vi "ParamClusterControlCore.vi"(7 "timeout in ms (100ms)":i32=100, 8 "IO queue":refnum<queue>, 9 "SetGetCommands":string[][](array[string]), 10 "Command queue":refnum<queue>, 11 "Cluster ref":refnum<vi>) -> ()   [LabVIEW 2021]
uses:
  <vilib>/Utility/Data Type/NI_Data Type.lvlib
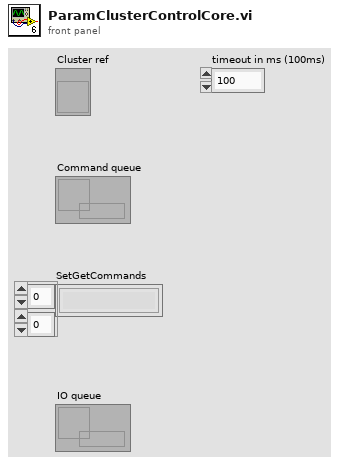
[diagram p1: front panel]
types:
  T1 = cluster{"Operation":enum16{"read", "write"}, "Data":string, "Queue":refnum<queue>}
  T2 = typedef "NI_Data Type.lvlib/Data Type.ctl" = enum8{"Invalid Type", "Void", "I8", "I16", "I32", "I64", "U8", "U16", "U32", "U64", "Single Float", "Double Float", "Extended Float", "Single Complex", "Double Complex", "Extended Complex", "Enum U8", "Enum U16", "Enum U32", "Enum U64", "Single Float With Unit", "Double Float With Unit", "Extended Float With Unit", "Single Complex with Unit", "Double Complex with Unit", "Extended Complex with Unit", "Boolean", "String", "Path", "Picture", "Tag", "Array", "Cluster", "Variant", "LV Variant", "Waveform", "Timestamp", "Digital Waveform", "Digital Data", "ExpressData", "Refnum", "External Data", "VI", "Poly VI", "LabVIEW Class Instance", "Fixed Point", "Set Collection", "Map Collection"}
  T3 = enum32{"Bad", "Idle", "Run top level", "Running"}
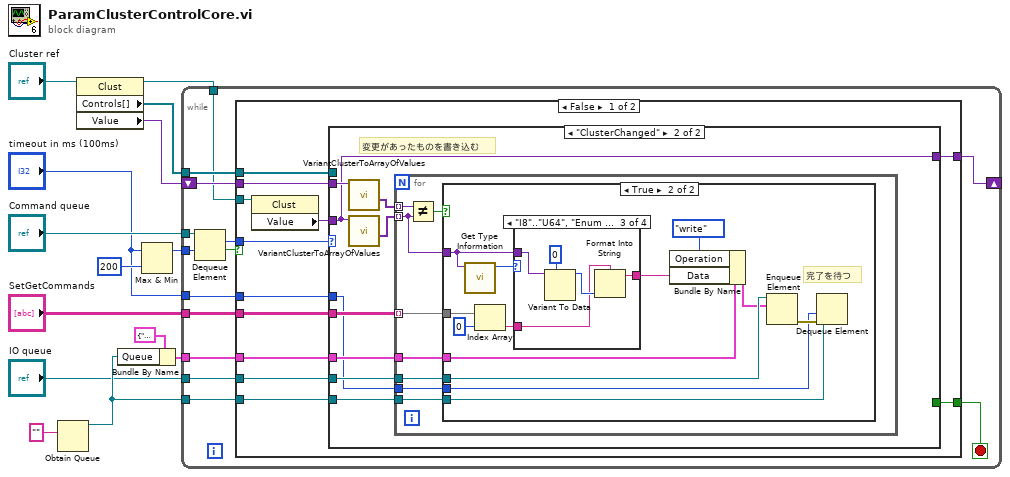
[diagram p0: block diagram]
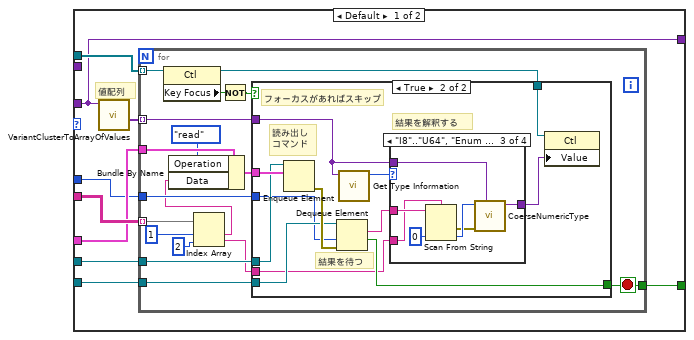
[diagram p2: hidden frame]
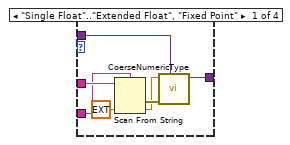
[diagram p4: hidden frame]
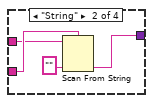
[diagram p5: hidden frame]
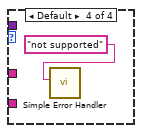
[diagram p6: hidden frame]
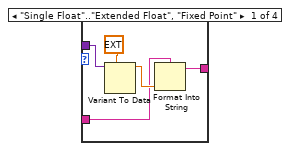
[diagram p8: hidden frame]
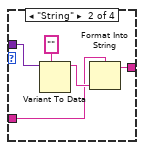
[diagram p9: hidden frame]
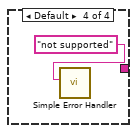
[diagram p10: hidden frame]
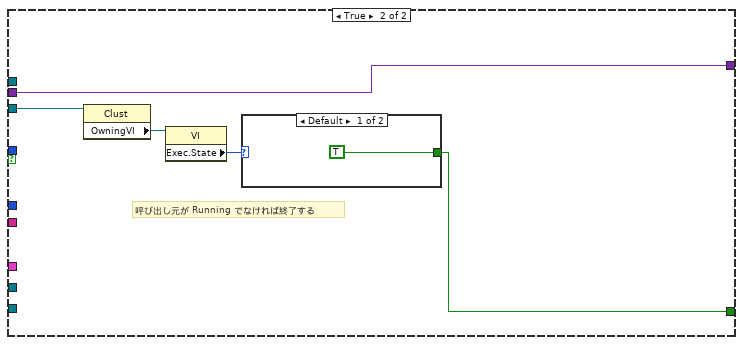
[diagram p11: hidden frame]
diagram:
  n1 = Obtain Queue(element data type="") -> (queue out=w8:refnum<queue>)  [unwired: 4 in, 2 out]
  n2 = property class="Clust"(reference="Cluster ref") -> (reference out=w3:refnum<vi>, "Controls[]"=w11:refnum<vi>[], "Value"=w9:variant)  [unwired: 1 in, 1 out]
  n3 = Bundle By Name(cluster=T1 {"Operation"=enum."read", "Data"="", "Queue"=refnum}, "Queue"=w8) -> (w7:T1)
  n4 = Max & Min(x="timeout in ms (100ms)", y=200 ("timeout in ms (-1)")) -> (max(x,y)=w5:i32)  [unwired: 1 out]
  n5 = while {
    tunnel: "Command queue" -> [w21]
    shift-right: [w23] -> _
    shift-left: w9 -> [w27]
    tunnel: "SetGetCommands" -> [w26]
    tunnel: "IO queue" -> [w25]
    tunnel: w8 -> [w24]
    tunnel: w11 -> [w19]
    tunnel: w3 -> [w18]
    tunnel: w5 -> [w17]
    tunnel: w7 -> [w16]
    tunnel: "timeout in ms (100ms)" -> [w15]
    stop <- w22 stop-if-true
    n6 = Dequeue Element(queue=w21, timeout in ms (-1)=w17) -> (element=w28:enum16{"UpdateCluster", "ClusterChanged"}, timed out?=w20:bool)  [unwired: 1 in, 2 out]
    n7 = case shown="False" w20 {
      tunnel: w28 -> [w33 _]
      tunnel: w27 -> [w40 w144]
      tunnel: w26 -> [w39 _]
      tunnel: w25 -> [w38 _]
      tunnel: w24 -> [w37 _]
      tunnel: [w36 w144] -> w23
      tunnel: [w35 w145] -> w22
      tunnel: w19 -> [w34 _]
      tunnel: w18 -> [w32 w148]
      tunnel: w16 -> [w30 _]
      tunnel: w15 -> [w29 _]
      frame False {
        n8 = property class="Clust"(reference=w32) -> ("Value"=w31:variant)  [unwired: 1 in, 2 out]
        n9 = case shown="\"ClusterChanged\"" w33 {
          tunnel: [w43 w100] -> w36
          tunnel: w40 -> [_ w106]
          tunnel: w39 -> [w48 w103]
          tunnel: w38 -> [w46 w102]
          tunnel: w37 -> [w47 w101]
          tunnel: [w44 _] -> w35
          tunnel: w34 -> [w45 _]
          tunnel: w31 -> [w43 w100]
          tunnel: w30 -> [w42 w99]
          tunnel: w29 -> [w41 w98]
          frame Default {
            # "値配列"
            n10 = call "VariantClusterToArrayOfValues.vi"("Cluster Variant"=w43) -> ("Values"=w49:variant[])  [unwired: 8 in, 2 out]
            n11 = for {
              tunnel: w49 -> [w62] mode=indexing
              tunnel: w48 -> [w61] mode=indexing
              tunnel: w47 -> [w63]
              tunnel: w46 -> [w64]
              tunnel: [w60] -> w44
              tunnel: w45 -> [w59] mode=indexing
              tunnel: w42 -> [w53]
              tunnel: w41 -> [w52]
              stop <- w60 stop-if-true
              n12 = property class="Ctl"(reference=w59) -> (reference out=w56:refnum<vi>, "Key Focus"=w57:bool)  [unwired: 1 in, 1 out]
              n13 = Index Array(array=w61, index #1=1 ("index"), index #2=2 ("index")) -> (element #1=w51:string, element #2=w54:string)
              n14 = Bundle By Name(cluster=w53, "Operation"=enum16{"read", "write"}."read", "Data"=w51) -> (w66:T1)
              n15 = Not(x=w57) -> (.not. x?=w58:bool)
              n16 = case shown="True" w58 {
                tunnel: w66 -> [_ w77]
                tunnel: w64 -> [_ w76]
                tunnel: w63 -> [_ w75]
                tunnel: w62 -> [_ w73]
                tunnel: [_ w71] -> w60
                tunnel: w56 -> [_ w70]
                tunnel: w54 -> [_ w68]
                tunnel: w52 -> [_ w67]
                frame False {
                }
                frame True {
                  # "フォーカスがあればスキップ"
                  # "結果を解釈する"
                  # "結果を待つ"
                  # "読み出し\nコマンド"
                  n17 = Enqueue Element(queue=w76, element=w77) -> (error out=w78:errorcluster)  [unwired: 2 in, 2 out]
                  n18 = Dequeue Element(queue=w75, timeout in ms (-1)=w67, error in (no error)=w78) -> (element=w72:string, timed out?=w71:bool)  [unwired: 2 out]
                  n19 = call <vilib>:"Get Type Information.vi"("variant"=w73) -> ("type"=w74:T2)  [unwired: 6 in, 4 out]
                  n20 = case shown="\"I8\"..\"U64\", \"Enum U8\"..\"Enum U64\"" w74 {
                    tunnel: w73 -> [w81 _ w92 _]
                    tunnel: w68 -> [w84 w88 w95 _]
                    tunnel: w72 -> [w85 w86 w96 _]
                    tunnel: [w80 w89 w91 _] -> w69
                    frame "Single Float".."Extended Float", "Fixed Point" {
                      n21 = Scan From String(format string=w84, input string=w85, default 1=ext 0.0 ("default value 1")) -> (error out=w83:errorcluster, output 1=w82:ext)  [unwired: 2 in, 2 out]
                      n22 = call "CoerseNumericType.vi"("Numeric Variant in"=w81, "error in (no error)"=w83, "Numeric"=w82) -> ("Numeric Variant out"=w80:variant)  [unwired: 7 in, 1 out]
                    }
                    frame "String" {
                      n23 = Scan From String(format string=w88, input string=w86, default 1="") -> (output 1=w89:string)  [unwired: 2 in, 3 out]
                    }
                    frame "I8".."U64", "Enum U8".."Enum U64" {
                      n24 = Scan From String(format string=w95, input string=w96, default 1=i64 0 ("default value 1")) -> (error out=w90:errorcluster, output 1=w93:i64)  [unwired: 2 in, 2 out]
                      n25 = call "CoerseNumericType.vi"("Numeric Variant in"=w92, "error in (no error)"=w90, "Numeric"=w93) -> ("Numeric Variant out"=w91:variant)  [unwired: 7 in, 1 out]
                    }
                    frame Default {
                      n26 = call <vilib>:"Simple Error Handler.vi"("error source (\" \")"="not supported" ("error source (\" \")")) -> ()  [unwired: 4 in, 5 out]
                    }
                  }
                  n27 = property class="Ctl"(reference=w70, "Value"=w69) -> ()  [unwired: 1 in, 2 out]
                }
              }
            }
          }
          frame "ClusterChanged" {
            # "変更があったものを書き込む"
            n28 = call "VariantClusterToArrayOfValues.vi"("Cluster Variant"=w106) -> ("Values"=w105:variant[])  [unwired: 8 in, 2 out]
            n29 = call "VariantClusterToArrayOfValues.vi"("Cluster Variant"=w100) -> ("Values"=w104:variant[])  [unwired: 8 in, 2 out]
            n30 = for {
              tunnel: w105 -> [w114] mode=indexing
              tunnel: w104 -> [w112] mode=indexing
              tunnel: w103 -> [w111] mode=indexing
              tunnel: w102 -> [w110]
              tunnel: w101 -> [w109]
              tunnel: w99 -> [w108]
              tunnel: w98 -> [w107]
              n31 = Not Equal?(x=w114, y=w112) -> (x != y?=w113:bool)
              n32 = case shown="True" w113 {
                tunnel: w112 -> [_ w124]
                tunnel: w111 -> [_ w125]
                tunnel: w110 -> [_ w122]
                tunnel: w109 -> [_ w118]
                tunnel: w108 -> [_ w117]
                tunnel: w107 -> [_ w116]
                frame False {
                }
                frame True {
                  # "完了を待つ"
                  n33 = call <vilib>:"Get Type Information.vi"("variant"=w124) -> ("type"=w127:T2)  [unwired: 6 in, 4 out]
                  n34 = Index Array(array=w125, index=0 ("index (row)")) -> (element=w123:string)
                  n35 = case shown="\"I8\"..\"U64\", \"Enum U8\"..\"Enum U64\"" w127 {
                    tunnel: w124 -> [w132 w137 w142 _]
                    tunnel: w123 -> [w129 w135 w140 _]
                    tunnel: [w128 w134 w139 _] -> w119
                    frame "Single Float".."Extended Float", "Fixed Point" {
                      n36 = Variant To Data(type=ext 0.0, Variant=w132) -> (data=w130:ext)  [unwired: 1 in, 1 out]
                      n37 = Format Into String(format string=w129, w130) -> (resulting string=w128:string)  [unwired: 2 in, 1 out]
                    }
                    frame "String" {
                      n38 = Variant To Data(type="", Variant=w137) -> (data=w136:string)  [unwired: 1 in, 1 out]
                      n39 = Format Into String(format string=w135, w136) -> (resulting string=w134:string)  [unwired: 2 in, 1 out]
                    }
                    frame "I8".."U64", "Enum U8".."Enum U64" {
                      n40 = Variant To Data(type=i64 0, Variant=w142) -> (data=w141:i64)  [unwired: 1 in, 1 out]
                      n41 = Format Into String(format string=w140, w141) -> (resulting string=w139:string)  [unwired: 2 in, 1 out]
                    }
                    frame Default {
                      n42 = call <vilib>:"Simple Error Handler.vi"("error source (\" \")"="not supported" ("error source (\" \")")) -> ()  [unwired: 4 in, 5 out]
                    }
                  }
                  n43 = Bundle By Name(cluster=w117, "Operation"=enum16{"read", "write"}."write", "Data"=w119) -> (w120:T1)
                  n44 = Enqueue Element(queue=w122, element=w120) -> (error out=w121:errorcluster)  [unwired: 2 in, 2 out]
                  n45 = Dequeue Element(queue=w118, timeout in ms (-1)=w116, error in (no error)=w121) -> ()  [unwired: 4 out]
                }
              }
            }
          }
        }
      }
      frame True {
        # "呼び出し元が Running でなければ終了する"
        n46 = property class="Clust"(reference=w148) -> ("OwningVI"=w147:refnum<vi>)  [unwired: 1 in, 2 out]
        n47 = property class="VI"(reference=w147) -> ("Exec.State"=w146:T3)  [unwired: 1 in, 2 out]
        n48 = case shown="Default" w146 {
          tunnel: [TRUE _] -> w145
          frame Default {
          }
          frame "Run top level", "Running" {
          }
        }
      }
    }
  }
